vi "close raw file ref.vi"() -> ()   [LabVIEW 2012]
panel:
  out "error out":errorcluster
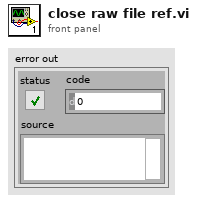
[diagram p1: front panel]
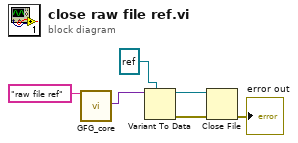
[diagram p0: block diagram]
diagram:
  n1 = call "GFG_core.vi"("Variable Name in"="raw file ref") -> ("Variant Out"=w5:variant)  [unwired: 12 in, 6 out]
  n2 = Variant To Data(type=refnum<file> refnum ("refnum out"), Variant=w5) -> (data=w2:refnum<file>, error out=w3:errorcluster)  [unwired: 1 in]
  n3 = Close File(refnum=w2, error in=w3) -> (error out=→"error out":errorcluster)  [unwired: 1 out]
